vi "LittleBoatHindbrainSense.vi"(8 "error in (no error)":errorcluster, 10 "Little Boat Queues":T1, 11 "connection ID":refnum<k16>) -> (0 "error out":errorcluster, 2 "UDP Time Out?":bool, 3 "connection ID out":refnum<k16>)   [LabVIEW 2013]
doc: "Code that processes the string sent from the camera processing code to tie the information back into our system."
uses:
  Data/TypeDefs/UTM Location.ctl
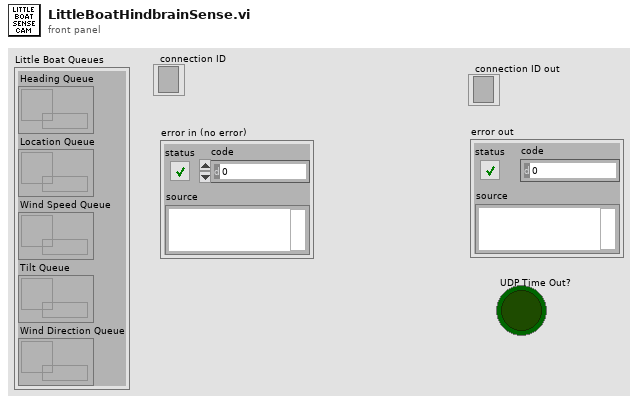
[diagram p1: front panel]
types:
  T1 = cluster{"Heading Queue":refnum<queue>, "Location Queue":refnum<queue>, "Wind Speed Queue":refnum<queue>, "Tilt Queue":refnum<queue>, "Wind Direction Queue":refnum<queue>}
  T2 = typedef "UTM Location.ctl" = cluster{"UTM Zone":dbl, "Hemisphere":enum16{"North", "South"}, "East":dbl, "North":dbl}
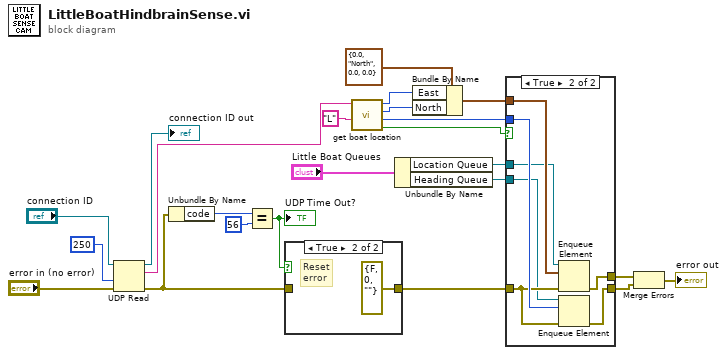
[diagram p0: block diagram]
diagram:
  n1 = UDP Read(connection ID="connection ID", timeout ms (25000)=250, 8:"error in (no error)") -> (data out=w6:string, error out=w7:errorcluster, 3:→"connection ID out":refnum<k16>)  [unwired: 1 in, 2 out]
  n2 = Unbundle By Name(w7) -> ("code"=w10:i32)
  n3 = Equal?(x=w10, y=56) -> (x = y?=w9:bool)
  "UDP Time Out?" <- w9
  n4 = case shown="True" w9 {
    tunnel: [w24 errorcluster {"status"=FALSE, "code"=0, "source"=""} ("error out")] -> w11
    tunnel: w7 -> [w24 _]
    frame False {
    }
    frame True {
      # "Reset\nerror"
    }
  }
  n5 = call "get boat location.vi"("Tug"="L", "Nav String"=w6) -> ("Valid ?"=w1:bool, "angle"=w2:i32, "y"=w3:i32, "x"=w4:i32)  [unwired: 6 in]
  n6 = Unbundle By Name("Little Boat Queues") -> ("Location Queue"=w17:refnum<queue>, "Heading Queue"=w16:refnum<queue>)
  n7 = Bundle By Name(cluster=T2 {"UTM Zone"=0.0, "Hemisphere"=enum."North", "East"=0.0, "North"=0.0} ("UTM Location"), "East"=w4, "North"=w3) -> (w18:T2)
  n8 = case shown="True" w1 {
    tunnel: [w26 w33] -> w23
    tunnel: [w26 w32] -> w22
    tunnel: w2 -> [_ w31]
    tunnel: w18 -> [_ w30]
    tunnel: w11 -> [w26 w29]
    tunnel: w17 -> [_ w28]
    tunnel: w16 -> [_ w27]
    frame False {
      # "if data invalid,\ndon't update\nqueues"
    }
    frame True {
      n9 = Enqueue Element(queue=w28, element=w30, error in (no error)=w29) -> (error out=w32:errorcluster)  [unwired: 1 in, 2 out]
      n10 = Enqueue Element(queue=w27, element=w31, error in (no error)=w29) -> (error out=w33:errorcluster)  [unwired: 1 in, 2 out]
    }
  }
  n11 = Merge Errors(w22, w23) -> (→"error out":errorcluster)
